vi "Textbox.vi"(7 "Message":string, 8 "error in (no error)":errorcluster, 9 "Textbox Location":T1, 10 "Textbox Name":string, 11 "ITX Commands in":refnum<class "ITX Commands.lvclass">) -> (0 "error out":errorcluster, 3 "ITX Commands out":refnum<class "ITX Commands.lvclass">)   [LabVIEW 2020, in "ITX Commands.lvclass"]
uses:
  ITX Commands.lvclass
  ITX Commands.lvclass/ITX Commands.ctl
panel:
  out "resulting string":string
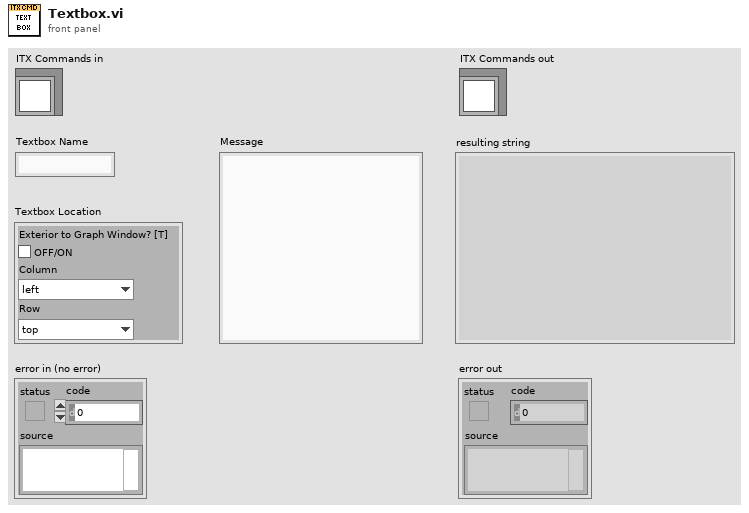
[diagram p1: front panel]
types:
  T1 = cluster{"Exterior to Graph Window? [T]":bool, "Column":enum16{"left", "middle", "right"}, "Row":enum16{"top", "center", "bottom"}}
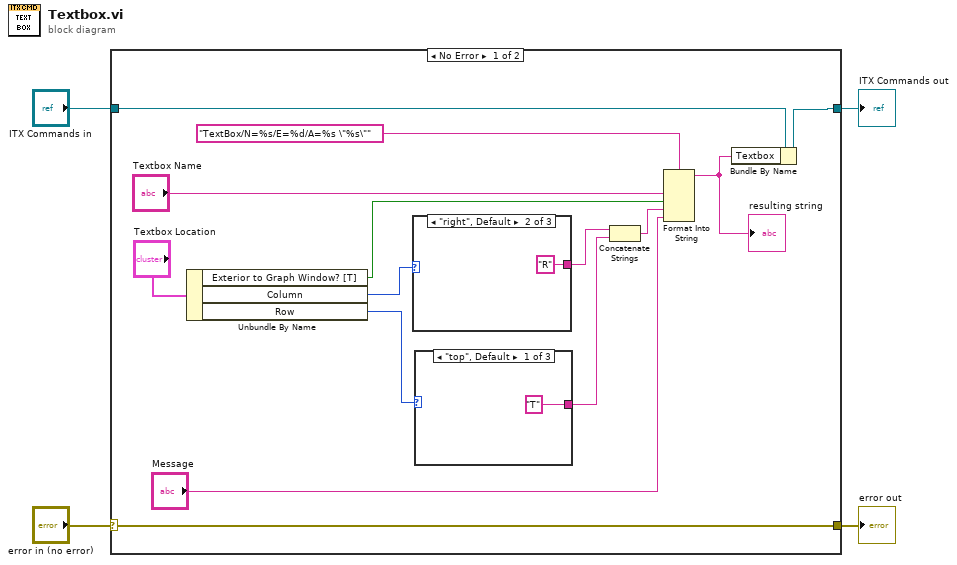
[diagram p0: block diagram]
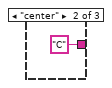
[diagram p2: hidden frame]
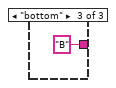
[diagram p3: hidden frame]
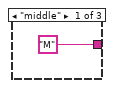
[diagram p4: hidden frame]
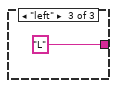
[diagram p5: hidden frame]
diagram:
  n1 = case shown="No Error" "error in (no error)" {
    selector: "error in (no error)" -> [w18 w26]
    tunnel: [w18 w26] -> w3
    tunnel: [w16 w25] -> w1
    tunnel: "ITX Commands in" -> [w17 w25]
    frame No Error {
      n2 = Unbundle By Name("Textbox Location") -> ("Exterior to Graph Window? [T]"=w12:bool, "Column"=w10:enum16{"left", "middle", "right"}, "Row"=w9:enum16{"top", "center", "bottom"})
      n3 = case shown="\"right\", Default" w10 {
        tunnel: ["M" "R" "L"] -> w8
        frame "middle" {
        }
        frame "right", Default {
        }
        frame "left" {
        }
      }
      n4 = case shown="\"top\", Default" w9 {
        tunnel: ["T" "C" "B"] -> w7
        frame "top", Default {
        }
        frame "center" {
        }
        frame "bottom" {
        }
      }
      n5 = Concatenate Strings(w8, w7) -> (w6:string)
      n6 = Format Into String(format string="TextBox/N=%s/E=%d/A=%s \"%s\"", "Textbox Name", w12, w6, "Message") -> (resulting string=w11:string)  [unwired: 2 in, 1 out]
      "resulting string" <- w11
      n7 = Bundle By Name(cluster=w17, "Textbox"=w11) -> (w16:refnum<class "ITX Commands.lvclass">)
    }
    frame Error {
    }
  }
  "error out" <- w3
  "ITX Commands out" <- w1
